vi "Write Charact Result.vi"(0 "Path in":refnum<class "Path.lvclass">, 11 "error in":errorcluster) -> (4 "Path out":refnum<class "Path.lvclass">, 15 "error out":errorcluster)   [LabVIEW 2023, in "RFFixtureCharact.Public.lvlib"]
uses:
  RFFixtureCharact.Public.lvlib
  Common/Base Classes/Path/Path.lvclass
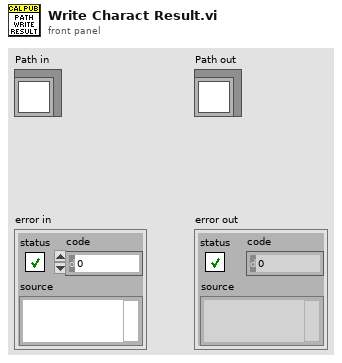
[diagram p1: front panel]
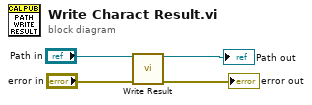
[diagram p0: block diagram]
diagram:
  n1 = call-dynamic "Write Result.vi"("Path in"="Path in", "error in (no error)"="error in") -> ("Path out"=→"Path out":refnum<class "Path.lvclass">, "error out"=→"error out":errorcluster)  [unwired: 12 in]
